vi "POV Control.vi"(1 "POV Number":dbl) -> ()   [LabVIEW 2018]
uses:
  Robot Global Data.vi
panel:
  out "Disc Collector Status":bool
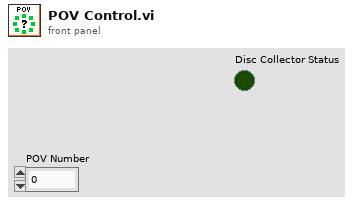
[diagram p1: front panel]
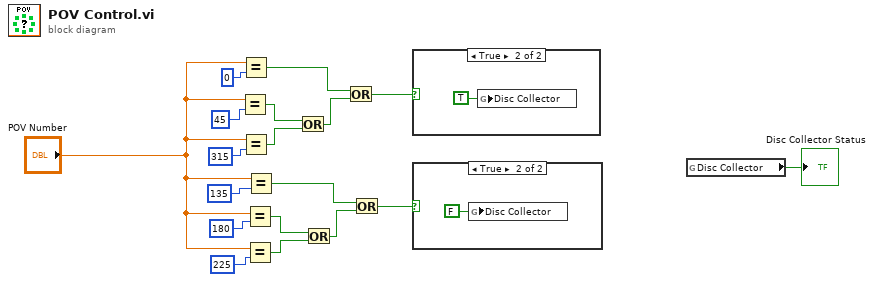
[diagram p0: block diagram]
diagram:
  n1 = Equal?(x="POV Number", y=45) -> (x = y?=w11:bool)
  n2 = Equal?(x="POV Number", y=0) -> (x = y?=w10:bool)
  n3 = Equal?(x="POV Number", y=315) -> (x = y?=w12:bool)
  n4 = Equal?(x="POV Number", y=180) -> (x = y?=w17:bool)
  n5 = Equal?(x="POV Number", y=225) -> (x = y?=w16:bool)
  n6 = Equal?(x="POV Number", y=135) -> (x = y?=w14:bool)
  n7 = Or(x=w11, y=w12) -> (x .or. y?=w13:bool)
  n8 = Or(x=w17, y=w16) -> (x .or. y?=w15:bool)
  n9 = Or(x=w10, y=w13) -> (x .or. y?=w6:bool)
  n10 = Or(x=w14, y=w15) -> (x .or. y?=w5:bool)
  n11 = case shown="True" w6 {
    frame False {
    }
    frame True {
      n12 = global write "Robot Global Data.vi" "Disc Collector"(TRUE ("Disc Collector")) -> ()
    }
  }
  n13 = case shown="True" w5 {
    frame False {
    }
    frame True {
      n14 = global write "Robot Global Data.vi" "Disc Collector"(FALSE ("Disc Collector")) -> ()
    }
  }
  n15 = global read "Robot Global Data.vi" "Disc Collector"() -> (→"Disc Collector Status":bool)
